vi "LINC CCSDS Callback.vi"(2 "command in":string, 3 "target name":string) -> (0 "command out":string, 1 "GUID":string)   [LabVIEW 2018, in "STEPkgDriver_LINC.lvlib"]
uses:
  STEPkgDriver_LINC.lvlib
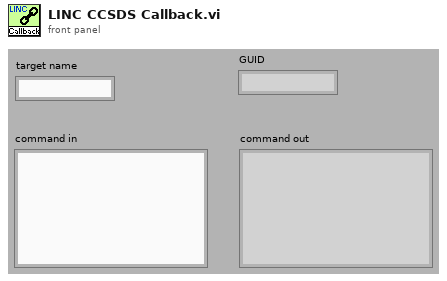
[diagram p1: front panel]
types:
  T1 = typedef "LVDateTimeRec.ctl" = cluster{"fractional second":dbl, "second":i32, "minute":i32, "hour":i32, "day of month":i32, "month":i32, "year":i32, "day of week":i32, "day of year":i32, "DST":i32}
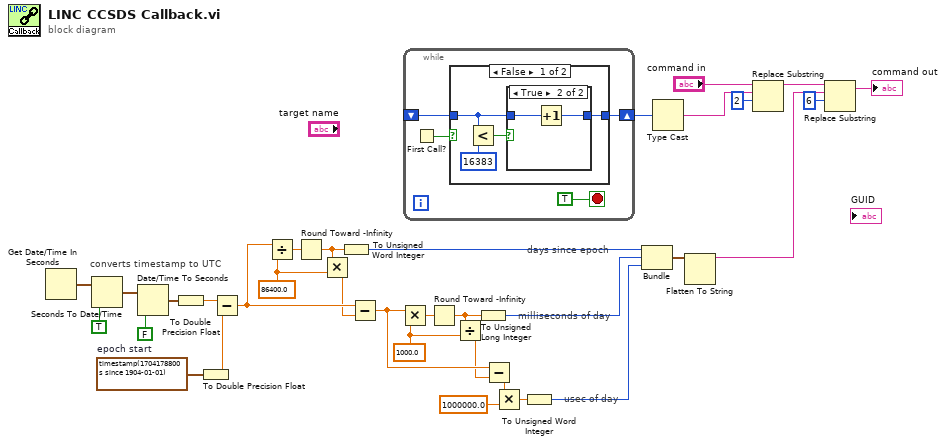
[diagram p0: block diagram]
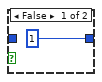
[diagram p2: hidden frame]
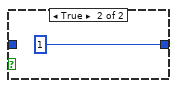
[diagram p3: hidden frame]
diagram:
  w15 = timestamp(1704178800 s since 1904-01-01)  # epoch start
  w25 = 1000.0 ("y")
  w29 = 86400.0 ("y")
  # "converts timestamp to UTC"
  # "usec of day"
  # "milliseconds of day"
  # "days since epoch"
  n1 = Get Date/Time In Seconds() -> (seconds since 1Jan1904=w3:timestamp)
  n2 = Seconds To Date/Time(time stamp (now)=w3, to UTC (F)=TRUE) -> (date time rec=w4:T1)
  n3 = Date/Time To Seconds(1:FALSE ("is UTC (F)"), 2:w4) -> (0:w2:timestamp)
  n4 = To Double Precision Float(number=w2) -> (double precision float=w1:dbl)
  n5 = To Double Precision Float(number=w15) -> (double precision float=w33:dbl)
  n6 = Subtract(x=w1, y=w33) -> (x-y=w31:dbl)
  n7 = Divide(x=w31, y=w29) -> (x/y=w32:dbl)
  n8 = Round Toward -Infinity(1:w32) -> (0:w30:dbl)
  n9 = Multiply(x=w30, y=w29) -> (x*y=w28:dbl)
  n10 = To Unsigned Word Integer(number=w30) -> (unsigned 16bit integer=w20:u16)
  n11 = Subtract(x=w31, y=w28) -> (x-y=w24:dbl)
  n12 = Multiply(x=w24, y=w25) -> (x*y=w27:dbl)
  n13 = while {
    shift-right: [w35] -> w12
    shift-left: _ -> [w34]
    stop <- TRUE stop-if-true
    n14 = First Call?() -> (First Call?: T/F=w36:bool)
    n15 = case shown="False" w36 {
      tunnel: [w38 u16 1] -> w35
      tunnel: w34 -> [w39 _]
      frame False {
        n16 = Less?(x=w39, y=u16 16383) -> (x < y?=w40:bool)
        n17 = case shown="True" w40 {
          tunnel: w39 -> [_ w44]
          tunnel: [u16 1 w43] -> w38
          frame False {
          }
          frame True {
            n18 = Increment(x=w44) -> (x+1=w43:u16)
          }
        }
      }
      frame True {
      }
    }
  }
  n19 = Round Toward -Infinity(1:w27) -> (0:w26:dbl)
  n20 = Divide(x=w26, y=w25) -> (x/y=w23:dbl)
  n21 = To Unsigned Long Integer(number=w26) -> (unsigned 32bit integer=w19:u32)
  n22 = Subtract(x=w24, y=w23) -> (x-y=w22:dbl)
  n23 = Multiply(x=w22, y=1000000.0) -> (x*y=w16:dbl)
  n24 = To Unsigned Word Integer(number=w16) -> (unsigned 16bit integer=w18:u16)
  n25 = Bundle(w20, w19, w18) -> (w17:cluster{u16, u32, u16})  [unwired: 1 out]
  n26 = Type Cast(x=w12) -> (*(type *) &x=w7:string)  [unwired: 1 in]
  n27 = Flatten To String(anything=w17) -> (data string=w8:string)  [unwired: 1 in, 4 out]
  n28 = Replace Substring(3:2 ("offset (0)"), 4:w7, 5:"command in") -> (1:w9:string)  [unwired: 2 out]
  n29 = Replace Substring(3:6 ("offset (0)"), 4:w8, 5:w9) -> (1:→"command out":string)  [unwired: 2 out]
